vi "5-Axis Servo Test Panel.vi"() -> ()   [LabVIEW 2014]
uses:
  EMC API/EMC_Typedef_Motor_Parameters.ctl
  Typedef/Typedef_Motor_Action.ctl
  Functional_Global/Typedef_FPGA_Interface_Action.ctl
  <vilib>/Motion/Express/_s/nimc.ex.clearFaults.clearFaults.axis.vi
  <vilib>/Motion/Express/_s/nimc.ex.power.power.axis.vi
  <vilib>/Motion/Express/_s/nimc.ex.resetPosition.resetPosition.axis.vi
  <vilib>/Utility/error.llb/Error Cluster From Error Code.vi
  <vilib>/rvi/errors/niLvFpgaAdjustHostInterfaceError.vi
  <vilib>/Motion/Express/_s/nimc.ex.read.readTrajectoryData.axis.vi
  <vilib>/Motion/Express/_s/nimc.ex.read.readMotionIO.axis.vi
  <vilib>/Motion/Express/_s/nimc.ex.findReferenceMove.startReferenceMove.axis.modeReverseLimit.vi
  <vilib>/Motion/Express/_s/nimc.ex.findReferenceMove.startReferenceMove.axis.modeHome.vi
  <vilib>/Motion/Express/_s/nimc.ex.findReferenceMove.startReferenceMove.axis.modeForwardLimit.vi
  <vilib>/Motion/BlockNode/FB.NIMotion.xnode
  <vilib>/rvi/interface/nirviReadWriteControl/nirviReadWriteControl.xnode
  <vilib>/rvi/interface/Simulation/niFpgaSimulationCallBeginRW.vi
  NiFpgaLv.dll
panel:
  in  "Reset Encoder 5":bool
  in  "Reset Encoder 4":bool
  in  "Reset Encoder 3":bool
  out "PID loop time (ticks)":u32=1994
  out "Position Feedback":i32[](array[numeric])
  out "AO Check":fxp<+/-,20,5>[](array[numeric])
  out "pos. error exceeded":bool[](array[boolean])
  out "pos. error":i16[](array[numeric])
  in  "Encoder filter value (us) Manual":u16=10
  in  "position error limit":i16=30000
  in  "AO Override?":bool
  in  "AO Manual":fxp<+/-,20,5>[](array[numeric])=[0.0, 0.0, 0.0, 0.0, 0.0]
  in  "Gains":T1(array[cluster])=[{"kp"=0.00341796875, "kd"=0.00146484375, "ki"=0.0}, {"kp"=0.00341796875, "kd"=0.00146484375, "ki"=0.0}, {"kp"=0.0, "kd"=0.0, "ki"=0.0}, {"kp"=0.0, "kd"=0.0, "ki"=0.0}, {"kp"=0.0, "kd"=0.0, "ki"=0.0}]
  in  "Limit Ranges":T2(array[cluster])=[{"output low"=-10.0, "output high"=10.0}, {"output low"=-10.0, "output high"=10.0}, {"output low"=0.0, "output high"=0.0}, {"output low"=0.0, "output high"=0.0}, {"output low"=0.0, "output high"=0.0}]
  in  "calls per sample (vel)":u16=40000
  in  "Reset Encoder 2":bool
  in  "Reset Encoder 1":bool
  in  "velocity":dbl=1000.0
  in  "Positions":dbl[](array[numeric])=[-5000.0, -5000.0, -5000.0, -5000.0, -5000.0, -5000.0]
  in  "resource":refnum<k21>="Axis 1"
  out "HOME active":bool
  out "REV active":bool
  out "FWD active":bool
  out "XY Graph":cluster{"X Array":dbl[], "Y Array":dbl[]}(graph)
  in  "interval":dbl=0.01 format="%#_13g"
  in  "Gear in/out":enum16{"Gear in", "Gear out"}(ring)
  in  "denominator":i32=1
  in  "numerator":i32=1
  in  "Master Axis":T3(ring)
  out "Array":dbl[](array[knob])=[0.0, 0.0, 0.0, 0.0, 0.0, 6.449939714304723] scale=0.0..1600.0
  in  "Clear Errors":bool
  in  "Command":T4
  in  "Motion Parameters":T5={"position"=1000.0, "velocity"=10000.0, "acceleration"=100000.0, "deceleration"=100000.0, "accel. jerk"=1000000.0, "decel. jerk"=1000000.0}
  in  "Axis Index":T3(ring)
  out "error":errorcluster
  in  "Stop all motors":bool
  in  "Execute Command":bool
  in  "stop":bool
  out "Axis Velocities":T6(graph)
  out "Axis Positions":T6(graph)
  # "Coordinate Move"
  # "Servo Parameters"
  # "Limit Switch Status"
  # "If position error exceeded:\n\n1. Set AO Override to T\n2. Set AO Manual to 0\n3. Reset encoder for that axis\n4. Reset RT traj to 0\n5. Set AO Override to F"
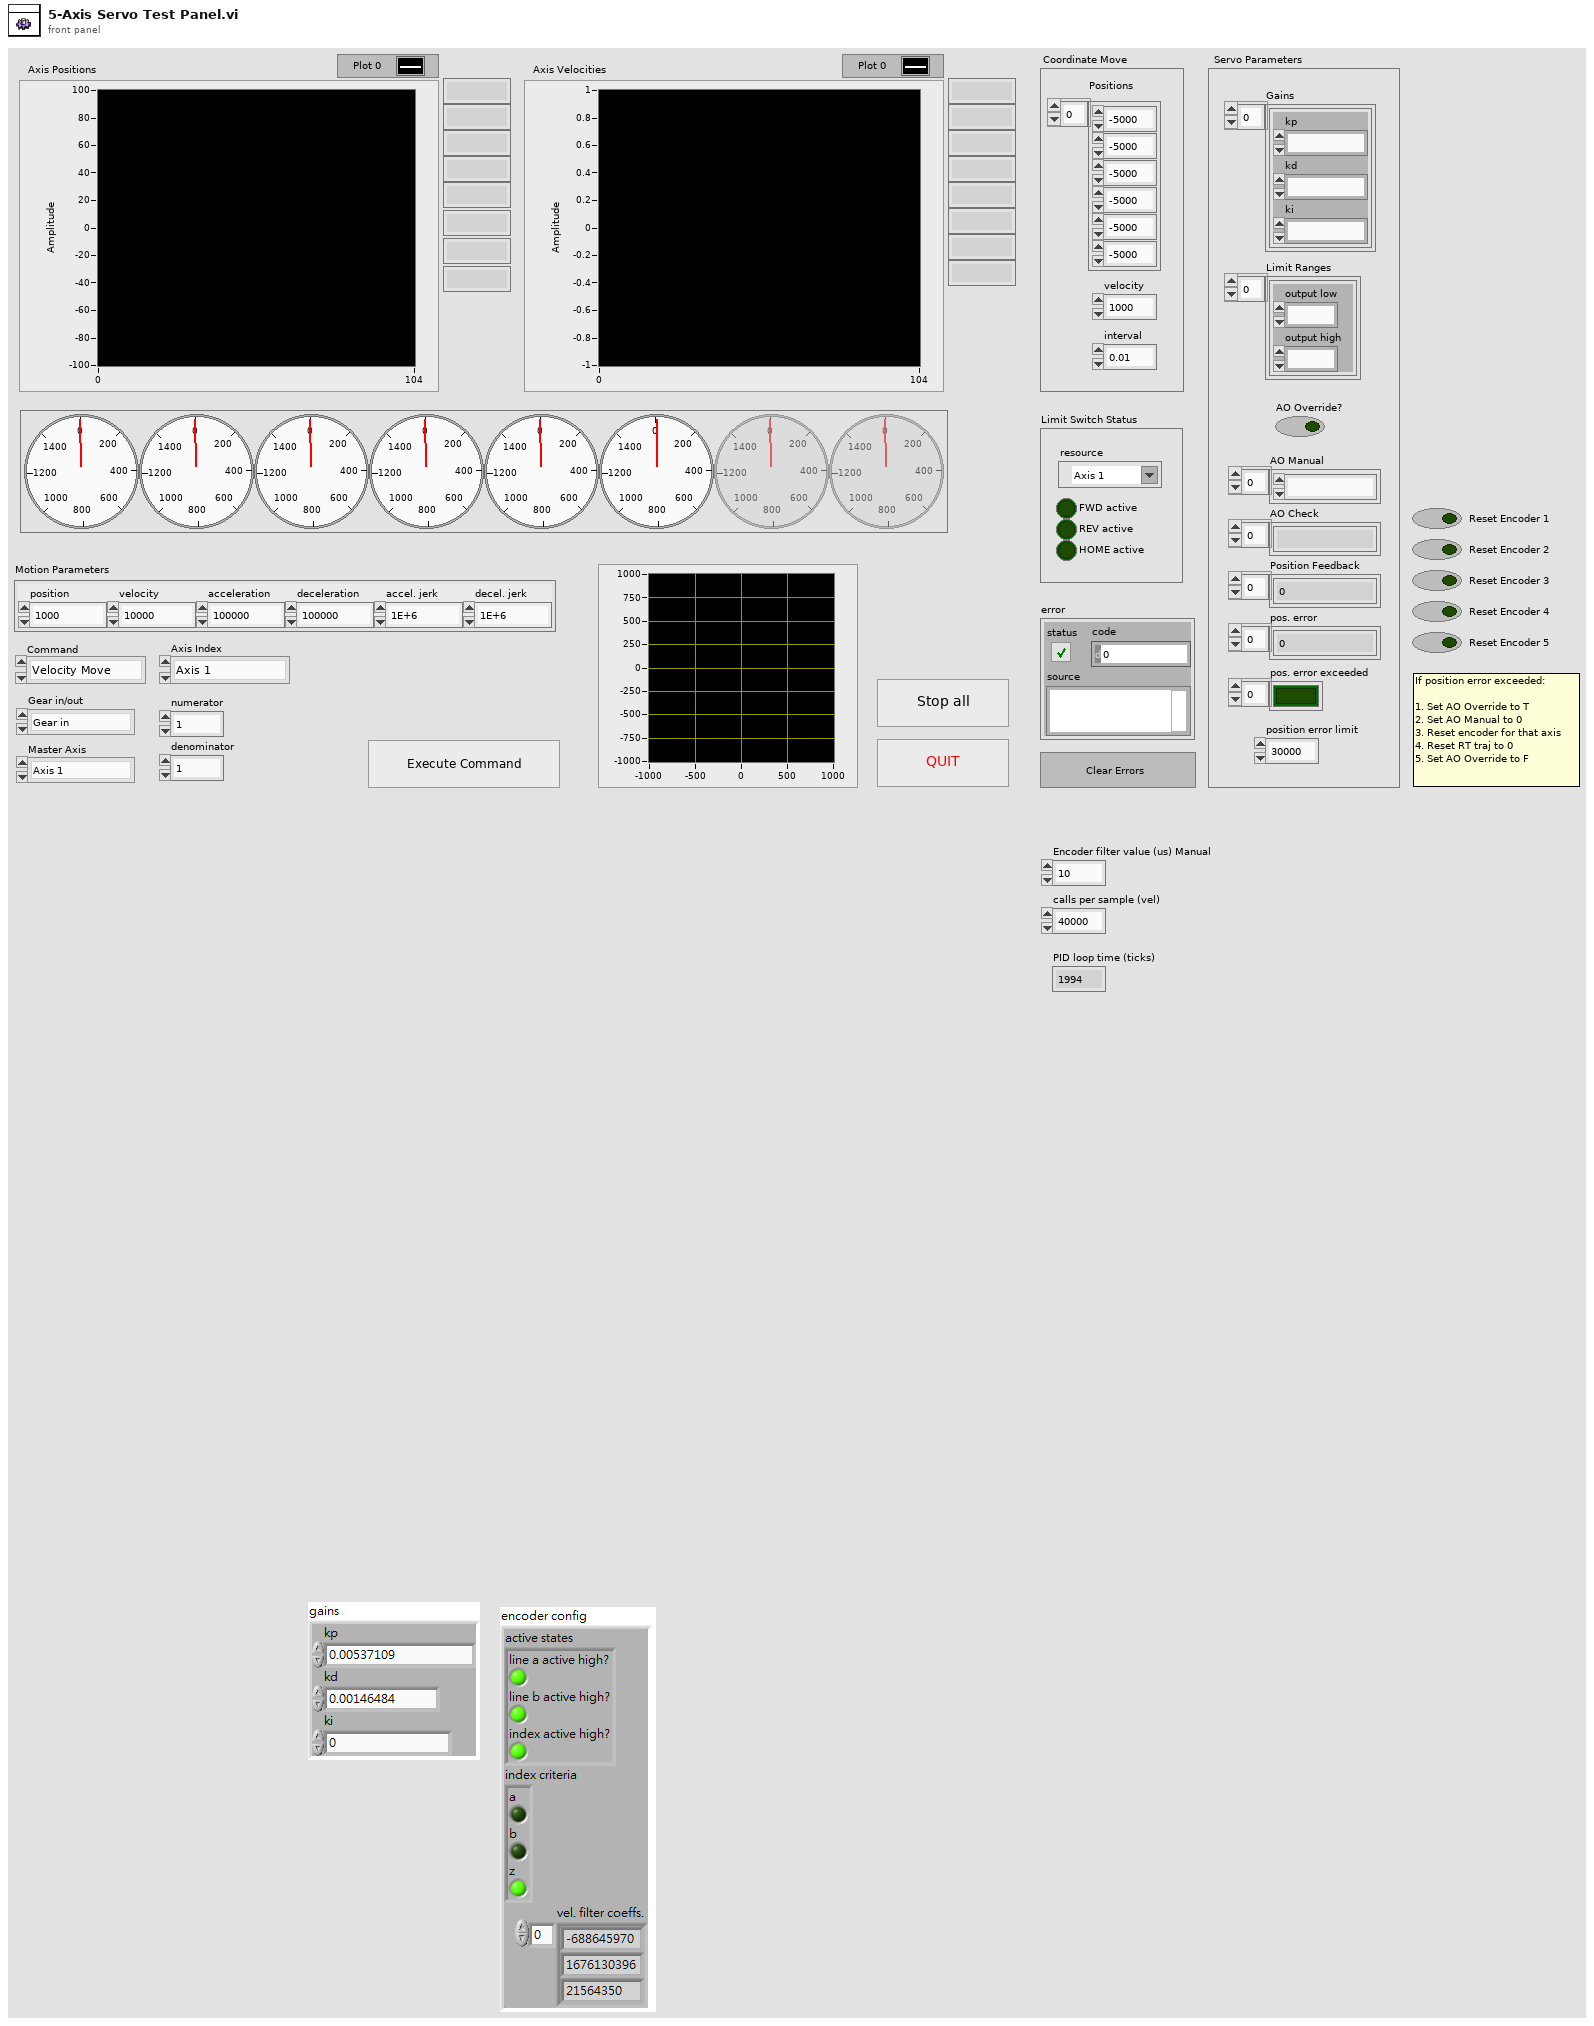
[diagram p1: front panel]
types:
  T1 = cluster{"kp":fxp<+,18,7>, "kd":fxp<+,18,7>, "ki":fxp<+,18,0>}[]
  T2 = cluster{"output low":fxp<+/-,18,6>, "output high":fxp<+/-,18,6>}[]
  T3 = enum16{"Axis 1", "Axis 2", "Axis 3", "Axis 4", "Axis 5", "Axis 6", "Axis 7", "Axis 8"}
  T4 = typedef "Typedef_Motor_Action.ctl" = enum16{"Velocity Move", "REL Pos Move", "ABS Pos Move", "Stop", "Reset Position", "Coordinate_move", "Contour_move", "Gearing", "Find Fwd Limit", "Find Rev Limit", "Find Home"}
  T5 = typedef "EMC_Typedef_Motor_Parameters.ctl" = cluster{"position":dbl, "velocity":dbl, "acceleration":dbl, "deceleration":dbl, "accel. jerk":dbl, "decel. jerk":dbl}
  T6 = cluster{"[0]":dbl, "[1]":dbl, "[2]":dbl, "[3]":dbl, "[4]":dbl, "[5]":dbl, "[6]":dbl, "[7]":dbl}
  T7 = typedef "Typedef_FPGA_Interface_Action.ctl" = enum16{"Initialize FPGA", "Get FPGA Reference", "Close FPGA"}
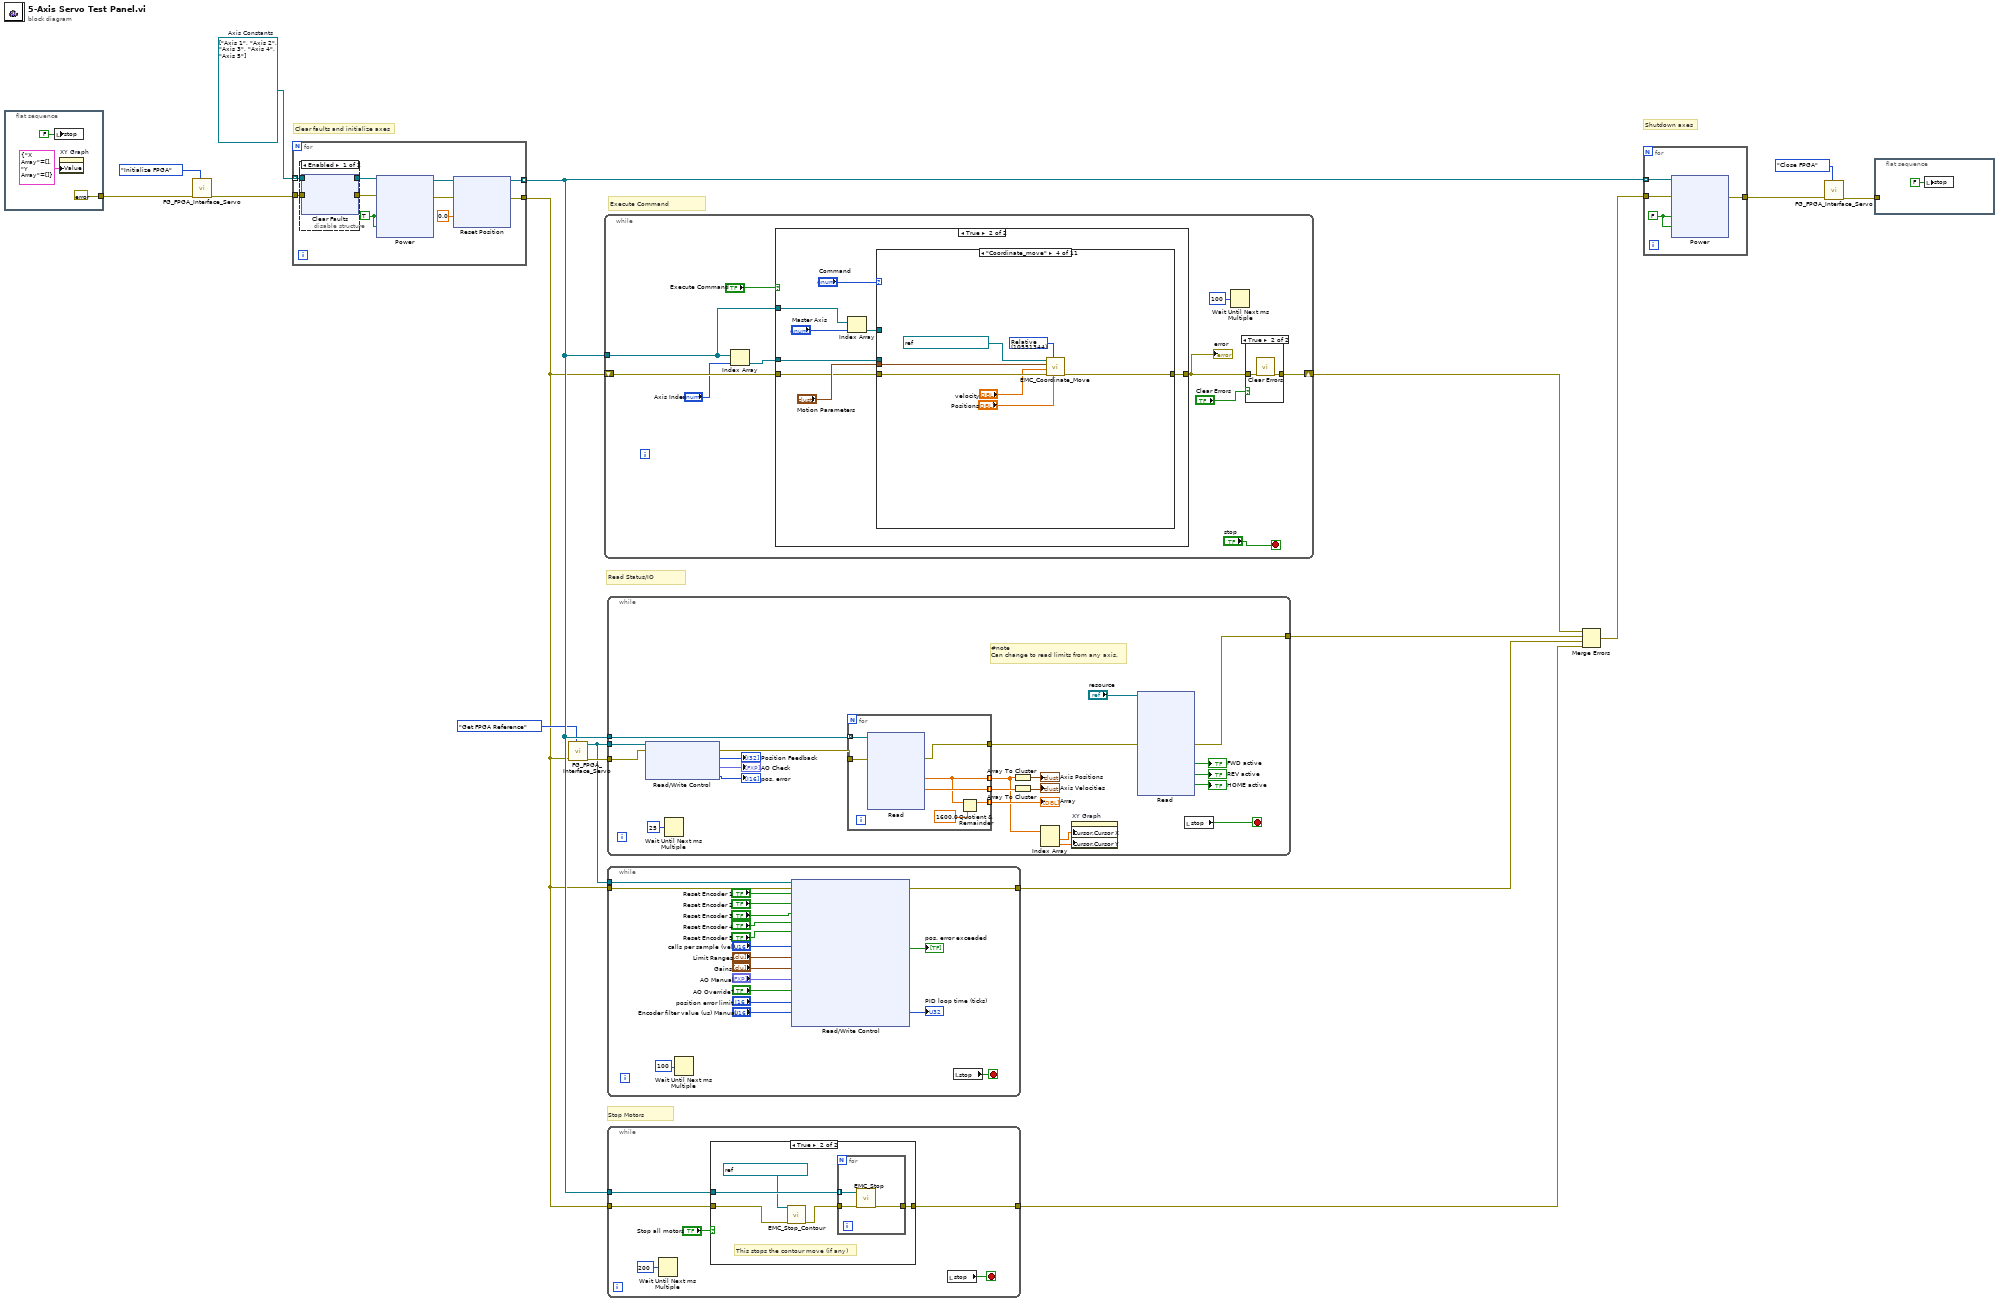
[diagram p0: block diagram]
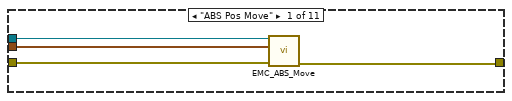
[diagram p6: hidden frame]
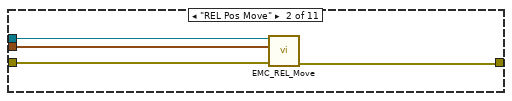
[diagram p7: hidden frame]
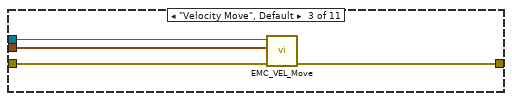
[diagram p8: hidden frame]
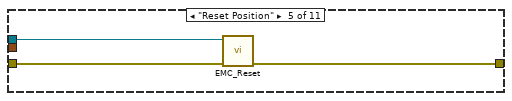
[diagram p9: hidden frame]
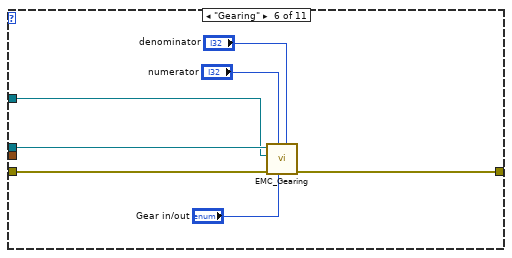
[diagram p10: hidden frame]
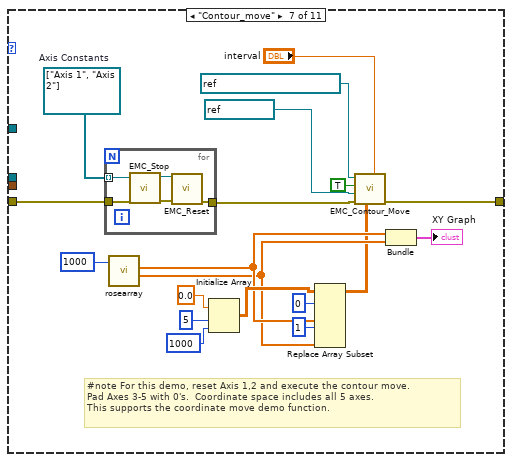
[diagram p11: hidden frame]
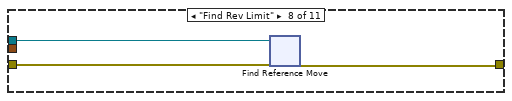
[diagram p12: hidden frame]
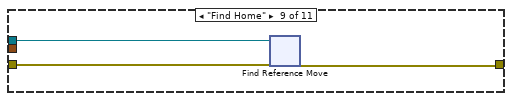
[diagram p13: hidden frame]
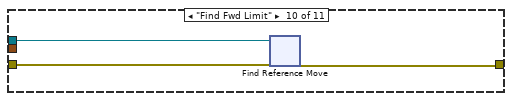
[diagram p14: hidden frame]
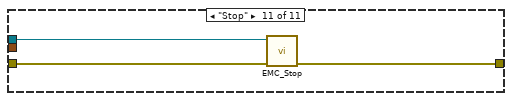
[diagram p15: hidden frame]
diagram:
  w17 = refnum<k21>[] ["Axis 1", "Axis 2", "Axis 3", "Axis 4", "Axis 5"]  # Axis Constants
  # "Read Status/IO"
  # "Clear faults and initialize axes"
  # "Shutdown axes"
  # "Execute Command"
  # "Stop Motors"
  n1 = flat-sequence {
    tunnel: [errorcluster {"status"=FALSE, "code"=0, "source"=""} ("error in (no error)")] -> w14
    frame #0 {
      n2 = local write "stop"(FALSE ("stop")) -> ()
      n3 = property on="XY Graph" class="XYGraph (strict)"("Value"=cluster{"X Array":dbl[], "Y Array":dbl[]} {"X Array"=[], "Y Array"=[]} ("XY Graph")) -> ()  [unwired: 2 in, 2 out]
    }
  }
  n4 = call "FG_FPGA_Interface_Servo.vi"("Action"=Typedef_FPGA_Interface_Action."Initialize FPGA", "error in"=w14) -> ("error out"=w11:errorcluster)  [unwired: 8 in, 1 out]
  n5 = for {
    tunnel: w17 -> [w24] mode=indexing
    tunnel: w11 -> [w23]
    tunnel: [w26] -> w6
    tunnel: [w25] -> w9 mode=indexing
    w30 = TRUE ("enable axis")
    n6 = disable-structure shown="Enabled" {
      disable-tunnel: w24 -> [w34 w40]
      disable-tunnel: w23 -> [w33 w39]
      disable-tunnel: [w32 w40] -> w22
      disable-tunnel: [w31 w39] -> w21
      frame Enabled {
        n7 = xnode ("Clear Faults")("resource"=w34, "error in"=w33) -> ("resource out"=w32:refnum<k21>, "error out"=w31:errorcluster)
      }
      frame Disabled {
      }
    }
    n8 = xnode ("Power")("enable axis"=w30, "enable drive"=w30, "resource"=w22, "error in"=w21) -> ("resource out"=w29:refnum<k21>, "error out"=w28:errorcluster)
    n9 = xnode ("Reset Position")("position"=0.0, "resource"=w29, "error in"=w28) -> ("resource out"=w25:refnum<k21>, "error out"=w26:errorcluster)
  }
  n10 = call "FG_FPGA_Interface_Servo.vi"("Action"=Typedef_FPGA_Interface_Action."Get FPGA Reference", "error in"=w6) -> ("error out"=w7:errorcluster, "FPGA VI Reference Out"=w1:refnum<k20>)  [unwired: 8 in]
  n11 = while {
    tunnel: w9 -> [w57]
    shift-right: [w58] -> w13
    shift-left: w6 -> [w62]
    stop <- "stop" stop-if-true
    n12 = Index Array(array=w57, index="Axis Index") -> (element=w63:refnum<k21>)
    n13 = case shown="True" "Execute Command" {
      tunnel: w62 -> [w69 w76]
      tunnel: w63 -> [_ w75]
      tunnel: [w69 w74] -> w59
      tunnel: w57 -> [_ w71]
      frame False {
      }
      frame True {
        n14 = Index Array(array=w71, index="Master Axis") -> (element=w70:refnum<k21>)
        n15 = case shown="\"Coordinate_move\"" "Command" {
          tunnel: "Motion Parameters" -> [w78 w82 w89 w90 _ _ _ _ _ _ _]
          tunnel: w76 -> [w81 w85 w88 w96 w98 w106 w118 w132 w151 w172 w192]
          tunnel: w75 -> [w79 w83 w87 _ w99 w105 _ w131 w150 w171 w190]
          tunnel: [w80 w84 w86 w95 w97 w104 w125 w133 w152 w173 w191] -> w74
          tunnel: w70 -> [_ _ _ _ _ w100 _ _ _ _ _]
          frame "ABS Pos Move" {
            n16 = call "EMC_ABS_Move.vi"("error in (no error)"=w81, "Motion Parameters"=w78, "axis"=w79) -> ("error out"=w80:errorcluster)  [unwired: 8 in]
          }
          frame "REL Pos Move" {
            n17 = call "EMC_REL_Move.vi"("error in (no error)"=w85, "Motion Parameters"=w82, "axis"=w83) -> ("error out"=w84:errorcluster)  [unwired: 8 in]
          }
          frame "Velocity Move", Default {
            n18 = call "EMC_VEL_Move.vi"("error in (no error)"=w88, "Motion Parameters"=w89, "axis"=w87) -> ("error out"=w86:errorcluster)  [unwired: 8 in]
          }
          frame "Coordinate_move" {
            w93 = 10551344 items=["Relative"=10551344, "Absolute"=10551337, "Relative To Capture"=10551345, "Velocity"=10551346, "Polyline"=11600101] ("line move mode")
            n19 = call "EMC_Coordinate_Move.vi"("position[]"="Positions", "line move mode"=w93, "error in (no error)"=w96, "velocity"="velocity", "Motion Parameters"=w90, "resource"=refnum<k21> "Coordinate Space 1") -> ("error out"=w95:errorcluster)  [unwired: 5 in]
          }
          frame "Reset Position" {
            n20 = call "EMC_Reset.vi"("error in (no error)"=w98, "axis"=w99) -> ("error out"=w97:errorcluster)  [unwired: 9 in]
          }
          frame "Gearing" {
            n21 = call "EMC_Gearing.vi"("denominator"="denominator", "Gear in/out"="Gear in/out", "numerator"="numerator", "error in (no error)"=w106, "master axis"=w100, "axis"=w105) -> ("error out"=w104:errorcluster)  [unwired: 5 in]
          }
          frame "Contour_move" {
            w116 = refnum<k21>[] ["Axis 1", "Axis 2"]  # Axis Constants
            # "#note For this demo, reset Axis 1,2 and execute the contour move.\nPad Axes 3-5 with 0's.  Coordinate space includes all 5 axes.\nThis supports the coordinate move demo function."
            n22 = for {
              tunnel: w118 -> [w129]
              tunnel: [w130] -> w117
              tunnel: w116 -> [w127] mode=indexing
              n23 = call "EMC_Stop.vi"("error in (no error)"=w129, "axis"=w127) -> ("error out"=w128:errorcluster, "axis out"=w126:refnum<k21>)  [unwired: 8 in]
              n24 = call "EMC_Reset.vi"("error in (no error)"=w128, "axis"=w126) -> ("error out"=w130:errorcluster)  [unwired: 9 in]
            }
            n25 = call "rosearray.vi"("Iterations"=u32 1000) -> ("Y Array"=w108:dbl[], "X Array"=w109:dbl[])  [unwired: 5 in, 1 out]
            n26 = Initialize Array(0.0 ("element"), 5 ("dimension size"), 1000 ("dimension size")) -> (w113:dbl[][])
            n27 = Replace Array Subset(array=w113, new element #1=w109, index (row) #1=0 ("index (row)"), new element #2=w108, index (row) #2=1 ("index (row)")) -> (w107:dbl[][])  [unwired: 2 in]
            n28 = call "EMC_Contour_Move.vi"("interval"="interval", "points[][]"=w107, "error in (no error)"=w117, "table"=refnum<k21> "Table 1" ("resource"), "overwrite"=TRUE, "coordinate"=refnum<k21> "Coordinate Space 1" ("resource")) -> ("error out"=w125:errorcluster)  [unwired: 5 in]
            n29 = Bundle("X Array"=w109, "Y Array"=w108) -> (→"XY Graph":cluster{"X Array":dbl[], "Y Array":dbl[]})  [unwired: 1 in]
          }
          frame "Find Rev Limit" {
            n30 = xnode "Find Reference Move"("resource"=w131, "error in"=w132) -> ("error out"=w133:errorcluster)  [unwired: 9 in, 2 out]
          }
          frame "Find Home" {
            n31 = xnode "Find Reference Move"("resource"=w150, "error in"=w151) -> ("error out"=w152:errorcluster)  [unwired: 11 in, 2 out]
          }
          frame "Find Fwd Limit" {
            n32 = xnode "Find Reference Move"("resource"=w171, "error in"=w172) -> ("error out"=w173:errorcluster)  [unwired: 9 in, 2 out]
          }
          frame "Stop" {
            n33 = call "EMC_Stop.vi"("error in (no error)"=w192, "axis"=w190) -> ("error out"=w191:errorcluster)  [unwired: 8 in, 1 out]
          }
        }
      }
    }
    "error" <- w59
    n34 = Wait Until Next ms Multiple(millisecond multiple=u32 100) -> ()  [unwired: 1 out]
    n35 = case shown="True" "Clear Errors" {
      tunnel: w59 -> [w66 w68]
      tunnel: [w66 w67] -> w58
      frame False {
      }
      frame True {
        n36 = call <vilib>:"Clear Errors.vi"("error in (no error)"=w68) -> ("error out"=w67:errorcluster)  [unwired: 5 in, 1 out]
      }
    }
  }
  n37 = while {
    tunnel: w7 -> [w195]
    tunnel: w9 -> [w211]
    tunnel: [w193] -> w16
    tunnel: w1 -> [w199]
    stop <- w200 stop-if-true
    # "#note \nCan change to read limits from any axis."
    n38 = xnode "Read/Write Control"("FPGA VI Reference In"=w199, "error in"=w195) -> ("error out"=w194:errorcluster, "Position Feedback"=→"Position Feedback":i32[], "AO Check"=→"AO Check":fxp<+/-,20,5>[], "pos. error"=→"pos. error":i16[])  [unwired: 1 out]
    n39 = Wait Until Next ms Multiple(millisecond multiple=u32 25) -> ()  [unwired: 1 out]
    n40 = for {
      tunnel: [w215] -> w202
      tunnel: [w216] -> w209 mode=indexing
      tunnel: [w217] -> w214 mode=indexing
      tunnel: w194 -> [w218]
      tunnel: w211 -> [w219] mode=indexing
      tunnel: [w220] -> w210 mode=indexing
      n41 = xnode ("Read")("resource"=w219, "error in"=w218) -> ("commanded position"=w216:dbl, "commanded vel."=w217:dbl, "error out"=w215:errorcluster)  [unwired: 2 out]
      n42 = Quotient & Remainder(x=w216, y=1600.0) -> (x-y*floor(x/y)=w220:dbl)  [unwired: 1 out]
    }
    "Array" <- w210
    n43 = Array To Cluster(array=w209) -> (cluster=→"Axis Positions":T6)
    n44 = Array To Cluster(array=w214) -> (cluster=→"Axis Velocities":T6)
    n45 = Index Array(array=w209) -> (element #1=w208:dbl, element #2=w207:dbl)  [unwired: 2 in]
    n46 = property on="XY Graph" class="XYGraph (strict)"("Cursor.Cursor X"=w208, "Cursor.Cursor Y"=w207) -> ()  [unwired: 2 in, 2 out]
    n47 = xnode ("Read")("resource"="resource", "error in"=w202) -> ("fwd. limit active"=→"FWD active":bool, "rev. limit active"=→"REV active":bool, "home active"=→"HOME active":bool, "error out"=w193:errorcluster)  [unwired: 6 out]
    n48 = local read "stop"() -> (w200:bool)
  }
  n49 = while {
    tunnel: w6 -> [w273]
    tunnel: w1 -> [w261]
    tunnel: [w260] -> w2
    stop <- w275 stop-if-true
    n50 = Wait Until Next ms Multiple(millisecond multiple=u32 100) -> ()  [unwired: 1 out]
    n51 = xnode "Read/Write Control"("FPGA VI Reference In"=w261, "error in"=w273, "Reset Encoder 1"="Reset Encoder 1", "Reset Encoder 2"="Reset Encoder 2", "Reset Encoder 3"="Reset Encoder 3", "Reset Encoder 4"="Reset Encoder 4", "Reset Encoder 5"="Reset Encoder 5", "calls per sample (vel)"="calls per sample (vel)", "Limit Ranges"="Limit Ranges", "Gains"="Gains", "AO Manual"="AO Manual", "AO Override?"="AO Override?", "position error limit"="position error limit", "Encoder filter value (us) Manual"="Encoder filter value (us) Manual") -> ("error out"=w260:errorcluster, "pos. error exceeded"=→"pos. error exceeded":bool[], "PID loop time (ticks)"=→"PID loop time (ticks)":u32)  [unwired: 2 out]
    n52 = local read "stop"() -> (w275:bool)
  }
  n53 = while {
    tunnel: w6 -> [w280]
    tunnel: w9 -> [w278]
    tunnel: [w276] -> w3
    stop <- w281 stop-if-true
    n54 = Wait Until Next ms Multiple(millisecond multiple=u32 200) -> ()  [unwired: 1 out]
    n55 = case shown="True" "Stop all motors" {
      tunnel: w280 -> [w282 w285]
      tunnel: [w282 w287] -> w276
      tunnel: w278 -> [_ w286]
      frame False {
      }
      frame True {
        # "This stops the contour move (if any)"
        n56 = call "EMC_Stop_Contour.vi"("error in (no error)"=w285, "coordinate"=refnum<k21> "Coordinate Space 1") -> ("error out"=w283:errorcluster)  [unwired: 9 in]
        n57 = for {
          tunnel: w283 -> [w290]
          tunnel: w286 -> [w288] mode=indexing
          tunnel: [w289] -> w287
          n58 = call "EMC_Stop.vi"("error in (no error)"=w290, "axis"=w288) -> ("error out"=w289:errorcluster)  [unwired: 8 in, 1 out]
        }
      }
    }
    n59 = local read "stop"() -> (w281:bool)
  }
  n60 = Merge Errors(w13, w16, w2, w3) -> (w10:errorcluster)
  n61 = for {
    tunnel: w9 -> [w294] mode=indexing
    tunnel: [w292] -> w12
    tunnel: w10 -> [w291]
    w293 = FALSE ("enable axis")
    n62 = xnode ("Power")("enable axis"=w293, "enable drive"=w293, "resource"=w294, "error in"=w291) -> ("error out"=w292:errorcluster)  [unwired: 1 out]
  }
  n63 = call "FG_FPGA_Interface_Servo.vi"("Action"=Typedef_FPGA_Interface_Action."Close FPGA", "error in"=w12) -> ("error out"=w15:errorcluster)  [unwired: 8 in, 1 out]
  n64 = flat-sequence {
    tunnel: w15 -> [_]
    frame #0 {
      n65 = local write "stop"(FALSE ("stop")) -> ()
    }
  }
